vi "RSNRPZ Chans Zeroing Complete State.vi"(8 "error in (no error)":errorcluster, 11 "VISA session":refnum<visa-resource-name> caption="VISA resource name") -> (0 "error out":errorcluster, 2 "Zeroing Completed":bool, 3 "dup VISA session":refnum<visa-resource-name> caption="VISA resource name")   [LabVIEW 2010]
doc: "This function should be used for polling whether a previously started zero calibration on a group of sensor has already finished. Zero calibration is an asynchronous operation and may take some seconds until completion. See the example code under RSNRPZ Channels Zero.vi on how to conduct a zeroing calibration on a group of sensors."
uses:
  rsnrpz_32.dll
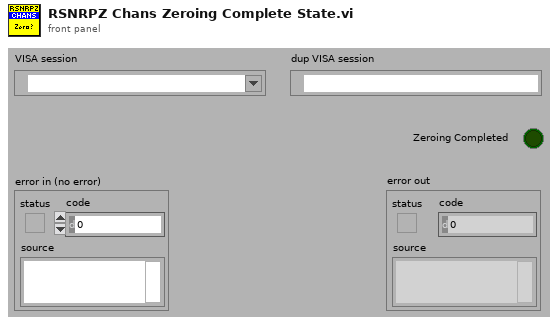
[diagram p1: front panel]
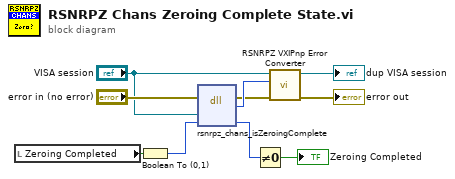
[diagram p0: block diagram]
diagram:
  n1 = local read "Zeroing Completed"() -> (w9:bool)
  n2 = Boolean To (0,1)(Boolean=w9) -> (0, 1=w7:i16)
  n3 = dll-call lib="rsnrpz_32.dll" fn="rsnrpz_chans_isZeroingComplete"(error in="error in (no error)", "VISA Session"="VISA session", "Zeroing Completed"=w7) -> (error out=w5:errorcluster, "Status"=w10:i32, "Zeroing Completed"=w8:u16)  [unwired: 3 in, 1 out]
  n4 = Not Equal To 0?(x=w8) -> (x != 0?=→"Zeroing Completed":bool)
  n5 = call <instrlib>:"RSNRPZ VXIPnp Error Converter.vi"("error in"=w5, "VXIPnp error code"=w10, "VISA session"="VISA session") -> ("error out"=→"error out":errorcluster, "dup VISA session"=→"dup VISA session":refnum<visa-resource-name>)  [unwired: 7 in]
